vi "DG5252.vi"() -> ()   [LabVIEW 2017]
panel:
  out "output control error":errorcluster
  out "configure error out":errorcluster
  in  "Output 2":bool
  in  "Output 1":bool
  in  "Waveform Function":u16(ring) items=["Sine", "Square", "Ramp", "Pulse", "Noise", "DC", "User"]
  in  "Channel Selection":u16(ring) items=["Channel 1", "Channel 2"]
  in  "Frequency (1000 Hz)":dbl=1000.0
  in  "Unit (0: Vpp)":u16(ring) items=["Vpp", "Vrms", "dB"]
  in  "DC Offset (0.00 V)":dbl
  in  "Amplitude (1)":dbl=1.0
  in  "?":bool
  in  "?":bool
  in  "VISA resource name":refnum<visa-resource-name>
  # "Rigol Technologies DG4/DG1Z General"
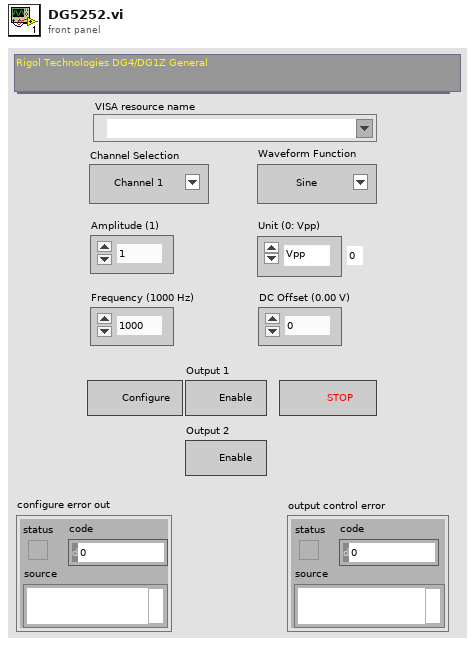
[diagram p1: front panel]
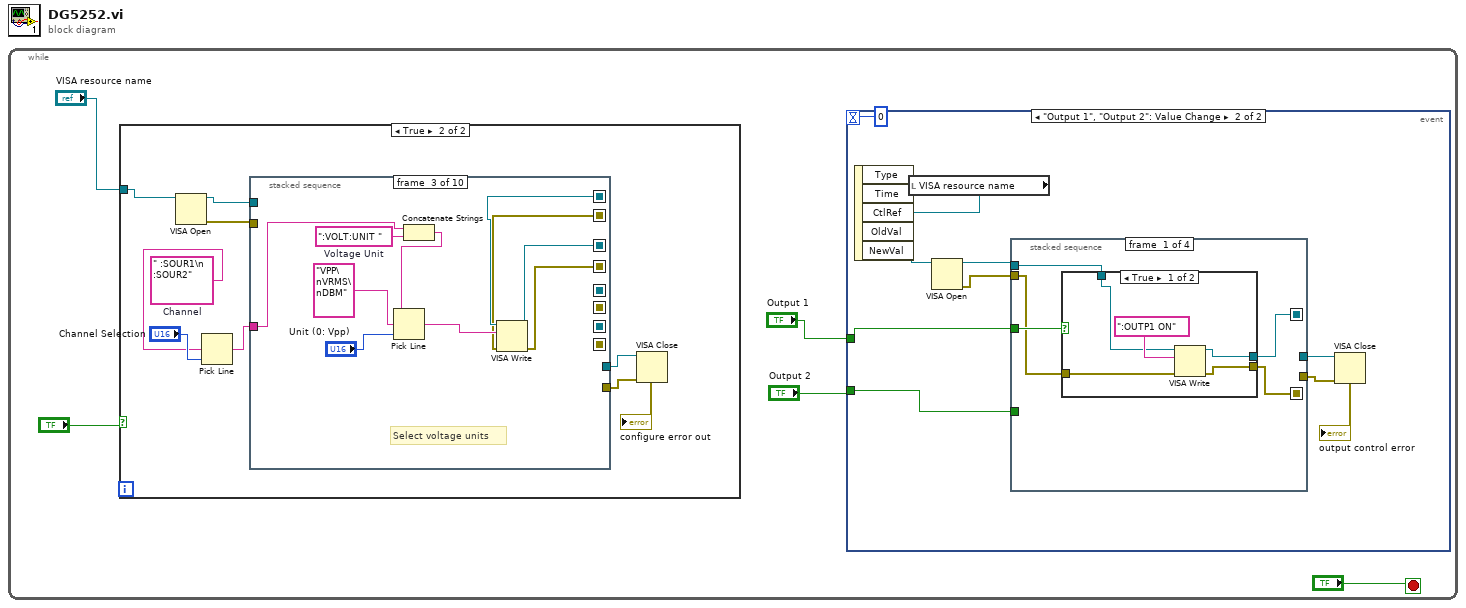
[diagram p0: block diagram]
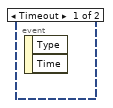
[diagram p2: hidden frame]
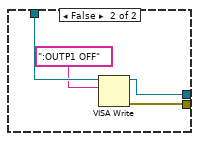
[diagram p3: hidden frame]
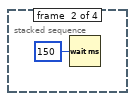
[diagram p4: hidden frame]
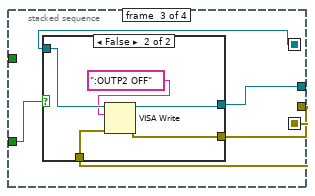
[diagram p5: hidden frame]
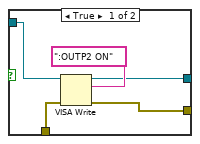
[diagram p6: hidden frame]
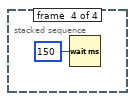
[diagram p7: hidden frame]
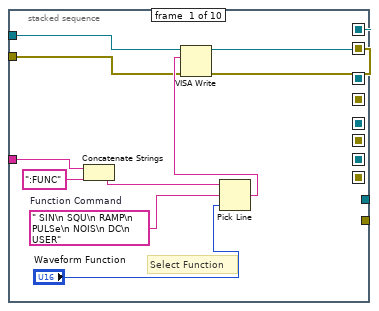
[diagram p9: hidden frame]
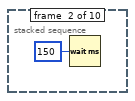
[diagram p10: hidden frame]
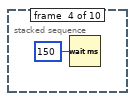
[diagram p11: hidden frame]
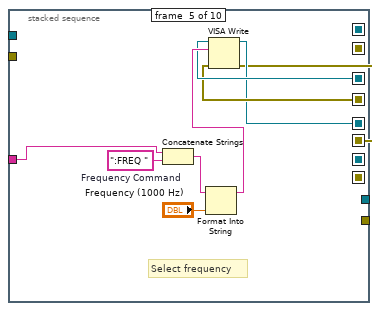
[diagram p12: hidden frame]
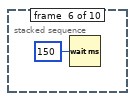
[diagram p13: hidden frame]
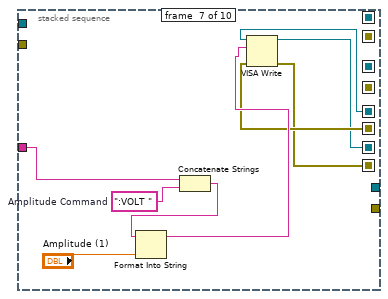
[diagram p14: hidden frame]
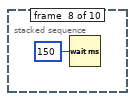
[diagram p15: hidden frame]
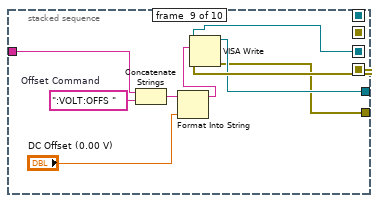
[diagram p16: hidden frame]
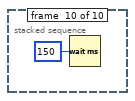
[diagram p17: hidden frame]
diagram:
  n1 = while {
    stop <- "?" stop-if-true
    n2 = case shown="True" "?" {
      tunnel: "VISA resource name" -> [_ w53]
      frame False {
      }
      frame True {
        w46 = " :SOUR1\n :SOUR2"  # Channel
        n3 = VISA Open(VISA resource name=w53) -> (VISA resource name=w52:refnum<visa-resource-name>, error out=w54:errorcluster)  [unwired: 4 in]
        n4 = Pick Line(multi-line string=w46, line index="Channel Selection") -> (output string=w48:string)  [unwired: 1 in]
        n5 = stacked-sequence {
          seq-local: [w58 _ _ _ _ _ _ _ _ _] -> [_ _ w70 _ _ _ _ _ _ _]
          seq-local: [w59 _ _ _ _ _ _ _ _ _] -> [_ _ w69 _ _ _ _ _ _ _]
          seq-local: [_ _ w68 _ _ _ _ _ _ _] -> [_ _ _ _ w81 _ _ _ _ _]
          seq-local: [_ _ w67 _ _ _ _ _ _ _] -> [_ _ _ _ w80 _ _ _ _ _]
          seq-local: [_ _ _ _ w79 _ _ _ _ _] -> [_ _ _ _ _ _ w91 _ _ _]
          seq-local: [_ _ _ _ w78 _ _ _ _ _] -> [_ _ _ _ _ _ w90 _ _ _]
          seq-local: [_ _ _ _ _ _ w89 _ _ _] -> [_ _ _ _ _ _ _ _ w101 _]
          seq-local: [_ _ _ _ _ _ w88 _ _ _] -> [_ _ _ _ _ _ _ _ w100 _]
          tunnel: w52 -> [w63 _ _ _ _ _ _ _ _ _]
          tunnel: w54 -> [w62 _ _ _ _ _ _ _ _ _]
          tunnel: [_ _ _ _ _ _ _ _ w99 _] -> w51
          tunnel: [_ _ _ _ _ _ _ _ w98 _] -> w50
          tunnel: w48 -> [w55 _ w66 _ w77 _ w87 _ w97 _]
          frame #0 {
            w57 = " SIN\n SQU\n RAMP\n PULSe\n NOIS\n DC\n USER"  # Function Command
            # "Select Function"
            n6 = Concatenate Strings(w55, ":FUNC" ("string (\"\")")) -> (w60:string)
            n7 = Pick Line(string ("")=w60, multi-line string=w57, line index="Waveform Function") -> (output string=w64:string)
            n8 = VISA Write(VISA resource name=w63, write buffer=w64, error in (no error)=w62) -> (VISA resource name out=w58:refnum<visa-resource-name>, error out=w59:errorcluster)  [unwired: 1 out]
          }
          frame #1 {
            n9 = Wait (ms)(milliseconds to wait=u32 150) -> ()  [unwired: 1 out]
          }
          frame #2 {
            w72 = ":VOLT:UNIT "  # Voltage Unit
            # "Select voltage units"
            n10 = Concatenate Strings(w66, w72) -> (w71:string)
            n11 = Pick Line(string ("")=w71, multi-line string="VPP\nVRMS\nDBM", line index="Unit (0: Vpp)") -> (output string=w74:string)
            n12 = VISA Write(VISA resource name=w70, write buffer=w74, error in (no error)=w69) -> (VISA resource name out=w68:refnum<visa-resource-name>, error out=w67:errorcluster)  [unwired: 1 out]
          }
          frame #3 {
            n13 = Wait (ms)(milliseconds to wait=u32 150) -> ()  [unwired: 1 out]
          }
          frame #4 {
            w83 = ":FREQ "  # Frequency Command
            # "Select frequency"
            n14 = Concatenate Strings(w77, w83) -> (w82:string)
            n15 = Format Into String(initial string=w82, "Frequency (1000 Hz)") -> (resulting string=w85:string)  [unwired: 2 in, 1 out]
            n16 = VISA Write(VISA resource name=w81, write buffer=w85, error in (no error)=w80) -> (VISA resource name out=w79:refnum<visa-resource-name>, error out=w78:errorcluster)  [unwired: 1 out]
          }
          frame #5 {
            n17 = Wait (ms)(milliseconds to wait=u32 150) -> ()  [unwired: 1 out]
          }
          frame #6 {
            w93 = ":VOLT "  # Amplitude Command
            n18 = Concatenate Strings(w87, w93) -> (w92:string)
            n19 = Format Into String(initial string=w92, "Amplitude (1)") -> (resulting string=w95:string)  [unwired: 2 in, 1 out]
            n20 = VISA Write(VISA resource name=w91, write buffer=w95, error in (no error)=w90) -> (VISA resource name out=w89:refnum<visa-resource-name>, error out=w88:errorcluster)  [unwired: 1 out]
          }
          frame #7 {
            n21 = Wait (ms)(milliseconds to wait=u32 150) -> ()  [unwired: 1 out]
          }
          frame #8 {
            w103 = ":VOLT:OFFS "  # Offset Command
            n22 = Concatenate Strings(w97, w103) -> (w102:string)
            n23 = Format Into String(initial string=w102, "DC Offset (0.00 V)") -> (resulting string=w105:string)  [unwired: 2 in, 1 out]
            n24 = VISA Write(VISA resource name=w101, write buffer=w105, error in (no error)=w100) -> (VISA resource name out=w99:refnum<visa-resource-name>, error out=w98:errorcluster)  [unwired: 1 out]
          }
          frame #9 {
            n25 = Wait (ms)(milliseconds to wait=u32 150) -> ()  [unwired: 1 out]
          }
        }
        n26 = VISA Close(VISA resource name=w51, error in (no error)=w50) -> (error out=→"configure error out":errorcluster)
      }
    }
    n27 = event shown="[1] \"Output 1\", \"Output 2\": Value Change" {
      selector: _ -> [_ _]
      dyn-events: _ -> [_ _]
      timeout: u32 0 ("Time") -> [_ _]
      tunnel: "Output 2" -> [_ w14]
      tunnel: "Output 1" -> [_ w13]
      event Timeout {
        n28 = event-data() -> ()  [unwired: 1 in, 2 out]
      }
      event "Output 1", "Output 2": Value Change {
        n29 = event-data() -> ()  [unwired: 1 in, 5 out]
        n30 = local read "VISA resource name"() -> (w12:refnum<visa-resource-name>)
        n31 = VISA Open(VISA resource name=w12) -> (VISA resource name=w11:refnum<visa-resource-name>, error out=w10:errorcluster)  [unwired: 4 in]
        n32 = stacked-sequence {
          seq-local: [w17 _ _ _] -> [_ _ w33 _]
          seq-local: [w15 _ _ _] -> [_ _ w31 _]
          tunnel: w11 -> [w19 _ _ _]
          tunnel: w14 -> [_ _ w34 _]
          tunnel: w13 -> [w18 _ _ _]
          tunnel: [_ _ w32 _] -> w9
          tunnel: w10 -> [w16 _ _ _]
          tunnel: [_ _ w30 _] -> w8
          frame #0 {
            n33 = case shown="True" w18 {
              tunnel: w19 -> [w23 w28]
              tunnel: [w22 w26] -> w17
              tunnel: w16 -> [w21 _]
              tunnel: [w20 w25] -> w15
              frame True {
                n34 = VISA Write(VISA resource name=w23, write buffer=":OUTP1 ON", error in (no error)=w21) -> (VISA resource name out=w20:refnum<visa-resource-name>, error out=w22:errorcluster)  [unwired: 1 out]
              }
              frame False {
                n35 = VISA Write(VISA resource name=w28, write buffer=":OUTP1 OFF") -> (VISA resource name out=w25:refnum<visa-resource-name>, error out=w26:errorcluster)  [unwired: 1 in, 1 out]
              }
            }
          }
          frame #1 {
            n36 = Wait (ms)(milliseconds to wait=u32 150) -> ()  [unwired: 1 out]
          }
          frame #2 {
            n37 = case shown="False" w34 {
              tunnel: w31 -> [w38 w44]
              tunnel: [w37 w42] -> w32
              tunnel: w33 -> [w36 w41]
              tunnel: [w35 w40] -> w30
              frame True {
                n38 = VISA Write(VISA resource name=w38, write buffer=":OUTP2 ON", error in (no error)=w36) -> (VISA resource name out=w35:refnum<visa-resource-name>, error out=w37:errorcluster)  [unwired: 1 out]
              }
              frame False {
                n39 = VISA Write(VISA resource name=w44, write buffer=":OUTP2 OFF", error in (no error)=w41) -> (VISA resource name out=w40:refnum<visa-resource-name>, error out=w42:errorcluster)  [unwired: 1 out]
              }
            }
          }
          frame #3 {
            n40 = Wait (ms)(milliseconds to wait=u32 150) -> ()  [unwired: 1 out]
          }
        }
        n41 = VISA Close(VISA resource name=w8, error in (no error)=w9) -> (error out=→"output control error":errorcluster)
      }
    }
  }
